vi "GUID.vi"() -> (3 "trimmed string":string caption="GUID")   [LabVIEW 2020]
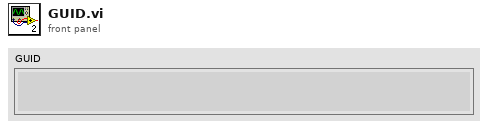
[diagram p1: front panel]
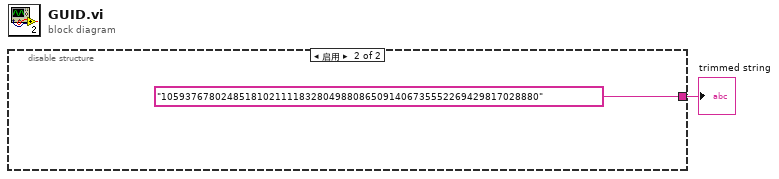
[diagram p0: block diagram]
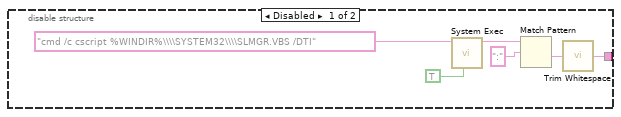
[diagram p2: hidden frame]
diagram:
  n1 = disable-structure shown="启用" {
    disable-tunnel: [w7 "105937678024851810211118328049880865091406735552269429817028880"] -> w1
    frame Disabled {
      n2 = call <vilib>:"System Exec.vi"("run minimized? (F)"=TRUE, "command line"="cmd /c cscript %WINDIR%\\\\SYSTEM32\\\\SLMGR.VBS /DTI") -> ("standard output"=w4:string)  [unwired: 6 in, 3 out]
      n3 = Match Pattern(string=w4, regular expression=":" ("正则表达式")) -> (after substring=w2:string)  [unwired: 1 in, 3 out]
      n4 = call <vilib>:"Trim Whitespace.vi"("string"=w2) -> ("trimmed string"=w7:string)  [unwired: 1 in]
    }
    frame Enabled {
    }
  }
  "trimmed string" <- w1
